vi "CODMn测量流程.vi"(11 "控制命令":T1(ring)) -> ()   [LabVIEW 2016, in "斯坦道CODMn.lvlib"]
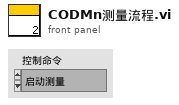
[diagram p1: front panel]
types:
  T1 = enum16{"启动测量", "标样核查", "零点核查", "跨度核查", "空白测试", "平行样测试", "加标回收", "空白校准", "标样校准", "初始化（清洗）", "停止测试", "仪器重启", "校时", "模式设置", "测量间隔设置"}
  T2 = cluster{"测量模式":enum16{"水样测量", "标样核查", "零点核查", "跨度核查", "空白测试", "加标回收", "平行样", "校零", "校标"}}
  T3 = enum16{"空闲", "水样测试", "标样核查", "零点核查", "跨度核查", "空白测试", "平行样测试", "质控样", "空白校准", "标样校准", "加标回收"}
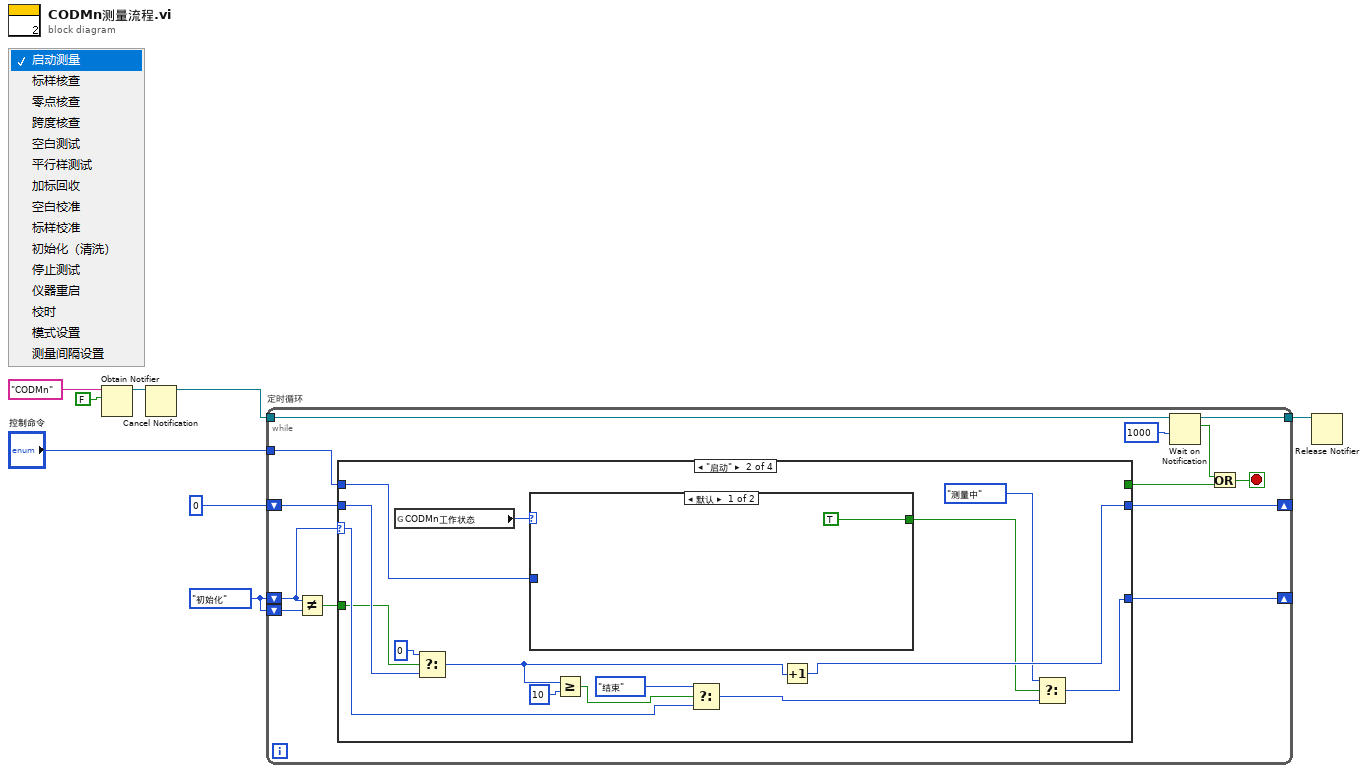
[diagram p0: block diagram]
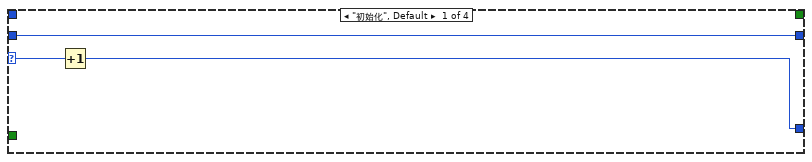
[diagram p2: hidden frame]
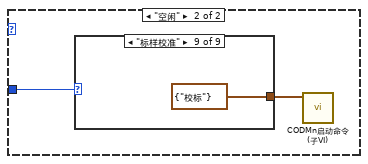
[diagram p3: hidden frame]
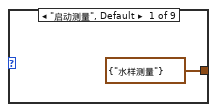
[diagram p4: hidden frame]
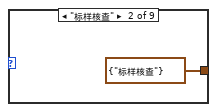
[diagram p5: hidden frame]
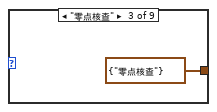
[diagram p6: hidden frame]
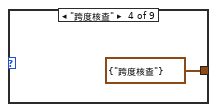
[diagram p7: hidden frame]
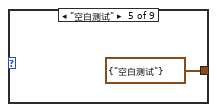
[diagram p8: hidden frame]
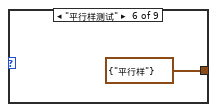
[diagram p9: hidden frame]
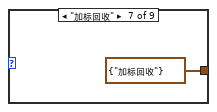
[diagram p10: hidden frame]
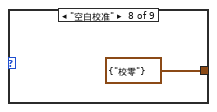
[diagram p11: hidden frame]
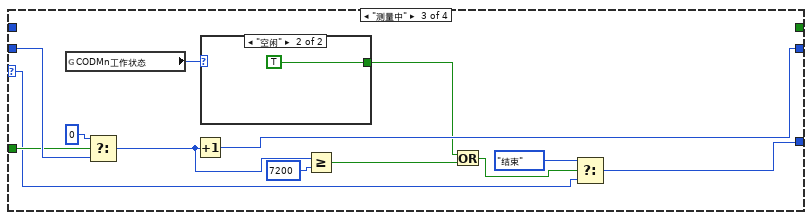
[diagram p12: hidden frame]
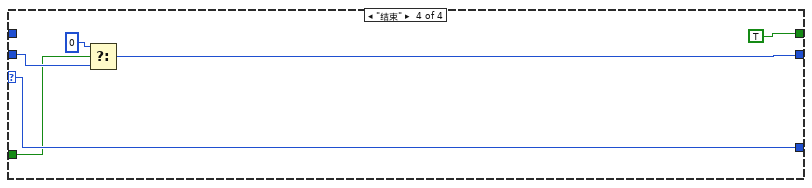
[diagram p14: hidden frame]
diagram:
  w1 = enum16{"初始化", "启动", "测量中", "结束"}."初始化"
  n1 = Obtain Notifier(name (unnamed)="CODMn" ("名称（未命名）"), notification data type=FALSE) -> (notifier out=w6:refnum<notifier>)  [unwired: 2 in, 2 out]
  n2 = Cancel Notification(0:w6) -> (8:w5:refnum<notifier>)  [unwired: 1 in, 2 out]
  n3 = while "定时循环" {
    tunnel: w5 -> [w21]
    tunnel: "控制命令" -> [w17]
    shift-right: [w16] -> _
    shift-left: w1 -> [w11]
    shift-right: [w14] -> _
    shift-left: 0 -> [w15]
    tunnel: [w12] -> w3
    shift-left: w1 -> [w10]
    stop <- w18 stop-if-true
    n4 = Not Equal?(x=w11, y=w10) -> (x != y?=w9:bool)
    n5 = case shown="\"启动\"" w11 {
      selector: w11 -> [w24 w33 w52 w71]
      tunnel: w17 -> [_ w39 _ _]
      tunnel: [w23 w28 w55 w71] -> w16
      tunnel: w15 -> [w22 w37 w63 w69]
      tunnel: [w22 w36 w62 w68] -> w14
      tunnel: [_ _ _ TRUE] -> w13
      tunnel: w9 -> [_ w30 w57 w66]
      frame "初始化", Default {
        n6 = Increment(x=w24) -> (x+1=w23:enum16{"初始化", "启动", "测量中", "结束"})
      }
      frame "启动" {
        n7 = global read "COD测量模式全局.vi" "CODMn工作状态"() -> (w31:T3)
        n8 = Select(t=0, s=w30, f=w37) -> (s? t:f=w35:i32)
        n9 = case shown="默认" w31 {
          tunnel: w39 -> [_ w42]
          tunnel: [TRUE _] -> w25
          frame Default {
          }
          frame "空闲" {
            n10 = case shown="\"标样校准\"" w42 {
              tunnel: [T2 {"测量模式"=enum."水样测量"} ("启动测量模式") T2 {"测量模式"=enum."标样核查"} ("启动测量模式") T2 {"测量模式"=enum."零点核查"} ("启动测量模式") T2 {"测量模式"=enum."跨度核查"} ("启动测量模式") T2 {"测量模式"=enum."空白测试"} ("启动测量模式") T2 {"测量模式"=enum."平行样"} ("启动测量模式") T2 {"测量模式"=enum."加标回收"} ("启动测量模式") T2 {"测量模式"=enum."校零"} ("启动测量模式") T2 {"测量模式"=enum."校标"} ("启动测量模式")] -> w41
              frame "启动测量", Default {
              }
              frame "标样核查" {
              }
              frame "零点核查" {
              }
              frame "跨度核查" {
              }
              frame "空白测试" {
              }
              frame "平行样测试" {
              }
              frame "加标回收" {
              }
              frame "空白校准" {
              }
              frame "标样校准" {
              }
            }
            n11 = call "CODMn启动命令 (子VI).vi"("启动测量模式"=w41) -> ()  [unwired: 11 in]
          }
        }
        n12 = Greater Or Equal?(x=w35, y=10) -> (x >= y?=w26:bool)
        n13 = Select(t=enum16{"初始化", "启动", "测量中", "结束"}."结束", s=w26, f=w33) -> (s? t:f=w29:enum16{"初始化", "启动", "测量中", "结束"})
        n14 = Increment(x=w35) -> (x+1=w36:i32)
        n15 = Select(t=enum16{"初始化", "启动", "测量中", "结束"}."测量中", s=w25, f=w29) -> (s? t:f=w28:enum16{"初始化", "启动", "测量中", "结束"})
      }
      frame "测量中" {
        n16 = global read "COD测量模式全局.vi" "CODMn工作状态"() -> (w58:T3)
        n17 = Select(t=0, s=w57, f=w63) -> (s? t:f=w61:i32)
        n18 = Increment(x=w61) -> (x+1=w62:i32)
        n19 = case shown="\"空闲\"" w58 {
          tunnel: [_ TRUE] -> w53
          frame Default {
          }
          frame "空闲" {
          }
        }
        n20 = Greater Or Equal?(x=w61, y=7200) -> (x >= y?=w56:bool)
        n21 = Or(x=w53, y=w56) -> (x .or. y?=w54:bool)
        n22 = Select(t=enum16{"初始化", "启动", "测量中", "结束"}."结束", s=w54, f=w52) -> (s? t:f=w55:enum16{"初始化", "启动", "测量中", "结束"})
      }
      frame "结束" {
        n23 = Select(t=0, s=w66, f=w69) -> (s? t:f=w68:i32)
      }
    }
    n24 = Wait on Notification(notifier=w21, timeout in ms (-1)=1000 ("超时毫秒(-1)")) -> (notifier out=w12:refnum<notifier>, notification=w19:bool)  [unwired: 2 in, 2 out]
    n25 = Or(x=w19, y=w13) -> (x .or. y?=w18:bool)
  }
  n26 = Release Notifier(notifier=w3) -> ()  [unwired: 2 in, 3 out]
